vi "writeU64FIFO.vi"(8 "error in (no error)":errorcluster, 9 "Timeout":i32, 10 "Data":u64[](array[numeric]), 11 "HealthAndStatusControlFIFO in":refnum<class "HealthAndStatusControlFIFO.lvclass">) -> (0 "error out":errorcluster, 2 "ElementsRemaining":u32, 3 "HealthAndStatusControlFIFO out":refnum<class "HealthAndStatusControlFIFO.lvclass">)   [LabVIEW 2016, in "HealthAndStatusControlFIFO.lvclass"]
uses:
  HealthAndStatusControlFIFO.lvclass
  HealthAndStatusControlFIFO.lvclass/HealthAndStatusControlFIFO.ctl
  FPGA/FPGA.lvclass
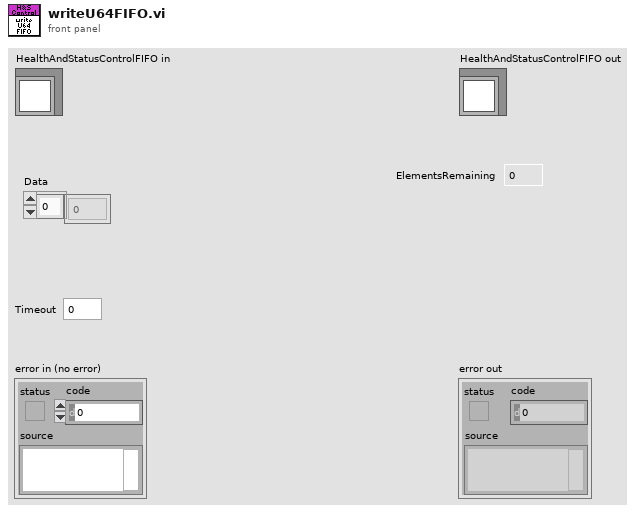
[diagram p1: front panel]
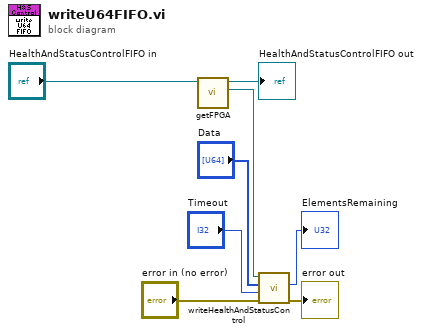
[diagram p0: block diagram]
diagram:
  n1 = call "getFPGA.vi"("HealthAndStatusControlFIFO in"="HealthAndStatusControlFIFO in") -> ("FPGA"=w6:refnum<class "FPGA.lvclass">, "HealthAndStatusControlFIFO out"=→"HealthAndStatusControlFIFO out":refnum<class "HealthAndStatusControlFIFO.lvclass">)  [unwired: 9 in]
  n2 = call "writeHealthAndStatusControl.vi"("error in (no error)"="error in (no error)", "Timeout"="Timeout", "Data"="Data", "FPGA in"=w6) -> ("error out"=→"error out":errorcluster, "ElementsRemaining"=→"ElementsRemaining":u32)  [unwired: 5 in, 1 out]
